vi "Create Path.vi"() -> (3 "Config File path":path)   [LabVIEW 2020, in "Config File Management.lvlib"]
doc: "Returns the path of the config file used for the vending maching configuration"
uses:
  Config File Management.lvlib
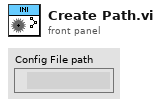
[diagram p1: front panel]
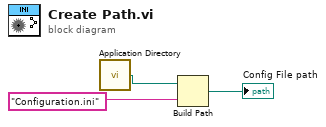
[diagram p0: block diagram]
diagram:
  n1 = call <vilib>:"Application Directory.vi"() -> ("Application Directory"=w3:path)
  n2 = Build Path(base path=w3, name or relative path="Configuration.ini") -> (appended path=→"Config File path":path)
